vi "AgNA_SetAttributeViInt32.vi"(7 "AttributeValue":i32 format="%.0g", 8 "error in (no error)":errorcluster {"code" format="%.0x"}, 9 "AttributeID":u32(ring)=1150002 items=["CHANNEL_AVERAGING_FACTOR"=1150002, "CHANNEL_MEASUREMENT_ELECTRICAL_DELAY_MEDIUM"=1150178, "CHANNEL_MEASUREMENT_ELECTRICAL_DELAY_UNITS"=1150175, "CHANNEL_MEASUREMENT_FORMAT"=1150014, "CHANNEL_MEASUREMENT_LIMIT_NUMBER"=1150020, "CHANNEL_MEASUREMENT_TIME_DOMAIN_GATING_SHAPE"=1150140, "CHANNEL_MEASUREMENT_TIME_DOMAIN_GATING_TYPE"=1150144, "CHANNEL_MEASUREMENT_TIME_DOMAIN_PARAMETERS"=1150137, "CHANNEL_MEASUREMENT_TIME_DOMAIN_TRANSFORM_MODE"=1150147, "CHANNEL_MEASUREMENT_TRACE_MATH"=1150017, "CHANNEL_POINTS"=1150007, "CHANNEL_SWEEP_MODE"=1150009, "CHANNEL_SWEEP_TYPE"=1150012, "CHANNEL_TRIGGER_MODE"=1150013, "DISPLAY_ARRANGE_WINDOWS"=1150181, "SYSTEM_TIME_OUT_MILLISECONDS"=1150040, "TRIGGER_SOURCE"=1150042, "WINDOW_SIZE"=1150133, "WINDOW_TABLE"=1150134], 10 "RepCapIdentifier":string, 11 "instrument handle":refnum<k15>) -> (0 "error out":errorcluster {"code" format="%.0x"}, 3 "instrument handle out":refnum<k15>)   [LabVIEW 2015]
uses:
  <instrlib>/Agilent NA/Agilent NA.lvlib
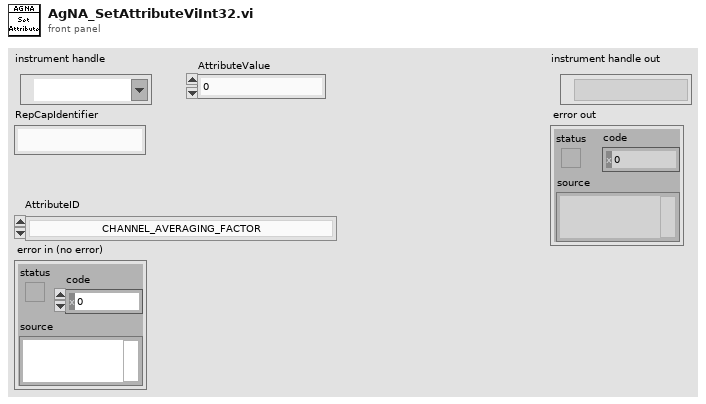
[diagram p1: front panel]
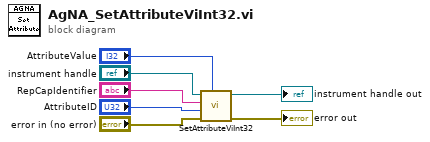
[diagram p0: block diagram]
diagram:
  n1 = call <instrlib>:"SetAttributeViInt32.vi"("AttributeValue"="AttributeValue", "error in (no error)"="error in (no error)", "AttributeID"="AttributeID", "RepCapIdentifier"="RepCapIdentifier", "instrument handle"="instrument handle") -> ("error out"=→"error out":errorcluster, "instrument handle out"=→"instrument handle out":refnum<k15>)  [unwired: 5 in]
